vi "Multi RefTriggerScope with digital read.vi"() -> ()   [LabVIEW 2023]
uses:
  RefTriggerApplication/ApplicationCluster.ctl
  <instrlib>/niScope/Controls/niScope trigger source digital.ctl
  <instrlib>/niScope/Controls/niScope trigger slope.ctl
  <instrlib>/niDigital/niDigital.llb/niDigital Export Signal.ctl
  <instrlib>/niDigital/niDigital.llb/niDigital Trigger Digital Edge - Edge.ctl
  <instrlib>/niDigital/niDigital.llb/niDigital Trigger Terminals.ctl
  <instrlib>/niDCPower/nidcpower.llb/niDCPower Export Signal - Signal.ctl
  <instrlib>/niDCPower/nidcpower.llb/niDCPower Wait For Event - Event.ctl
  <instrlib>/niScope/Configure/Trigger/niScope Configure Trigger Digital.vi
  <instrlib>/niDigital/niDigital.llb/niDigital Disable Start Trigger.vi
  <instrlib>/niDigital/niDigital.llb/niDigital Configure Digital Edge Start Trigger.vi
  <instrlib>/niScope/Acquire/Fetch/niScope Fetch.vi
panel:
  out "SMU":dbl[](graph)
  in  "Trigger Through":enum16{"DigitalPattern", "SMU"}(ring)
  in  "Instrument Settings":enum32{"SMU", "Scope", "Digital Pattern"}(tab)
  in  "SMU name":refnum<k15>
  in  "Scope Name 2":refnum<k15>="Scope_5152_C02_S05" caption="Scope  Name(s)"
  in  "Scope Name":refnum<k15>="Scope_5152_C02_S05" caption="Scope  Name(s)"
  in  "Sample Rate":dbl=5000000.0 format="%#.2p"
  in  "Record Length":i32=10000 format="%.0p"
  in  "Reference Position":dbl=50.0 caption="Ref Position" format="%#.1f"
  in  "DigiPat name":refnum<k15>
  in  "pin list":string="SPICLock, SPIData"
  out "Scope":dbl[][](graph)
  out "Digital Data":u32[][](array[numeric])
  out "error out":errorcluster
  in  "error in":errorcluster
  # "SDA"
  # "Other pin"
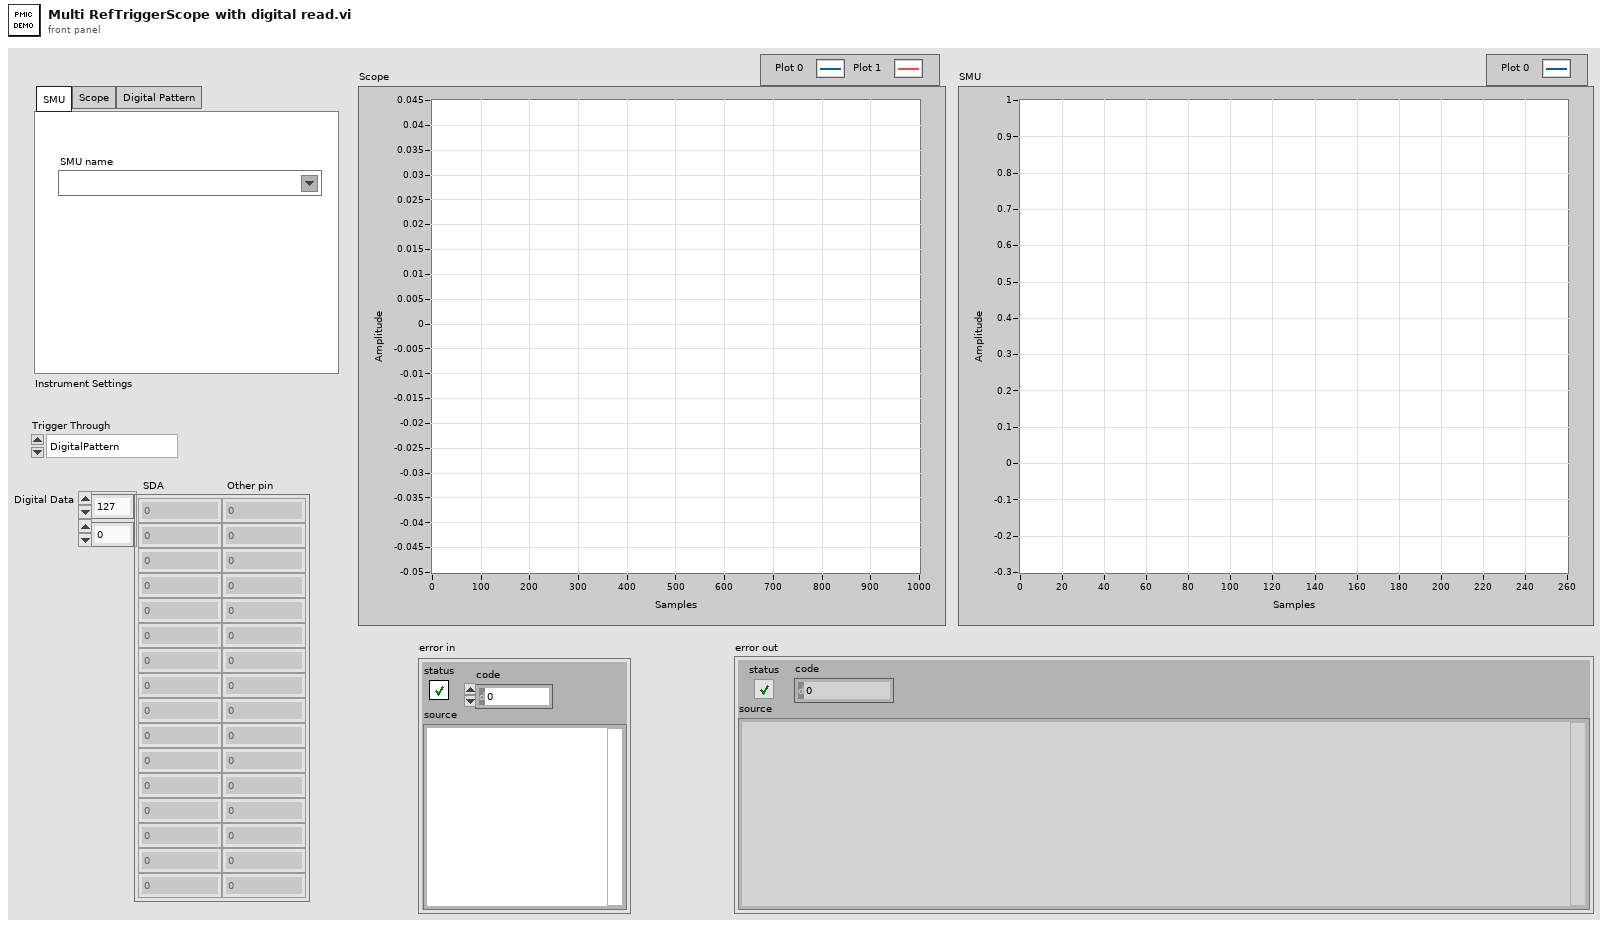
[diagram p1: front panel]
types:
  T1 = typedef "ApplicationCluster.ctl" = cluster{"Scope Name":refnum<k15>, "Scope channel name":string, "DigiPat name":refnum<k15>, "pin list":string, "DigitalWaveformName":string, "DigitalData":u32[][], "SMU name":refnum<k15>, "SMU Channel Name":string, "SMU Sequence Name":string, "Scope wfm":dbl[][], "SMU wfv":dbl[], "Record Length Scope":i32, "Scope Name 2":refnum<k15>, "Scope channel name 2":string}
  T2 = typedef "niScope trigger source digital.ctl" = string
  T3 = typedef "niDigital Trigger Terminals.ctl" = string
  T4 = typedef "niScope trigger slope.ctl" = i32
  T5 = typedef "niDigital Export Signal.ctl" = i32
  T6 = typedef "niDCPower Export Signal - Signal.ctl" = i32
  T7 = typedef "niDigital Trigger Digital Edge - Edge.ctl" = i32
  T8 = typedef "niDCPower Wait For Event - Event.ctl" = i32
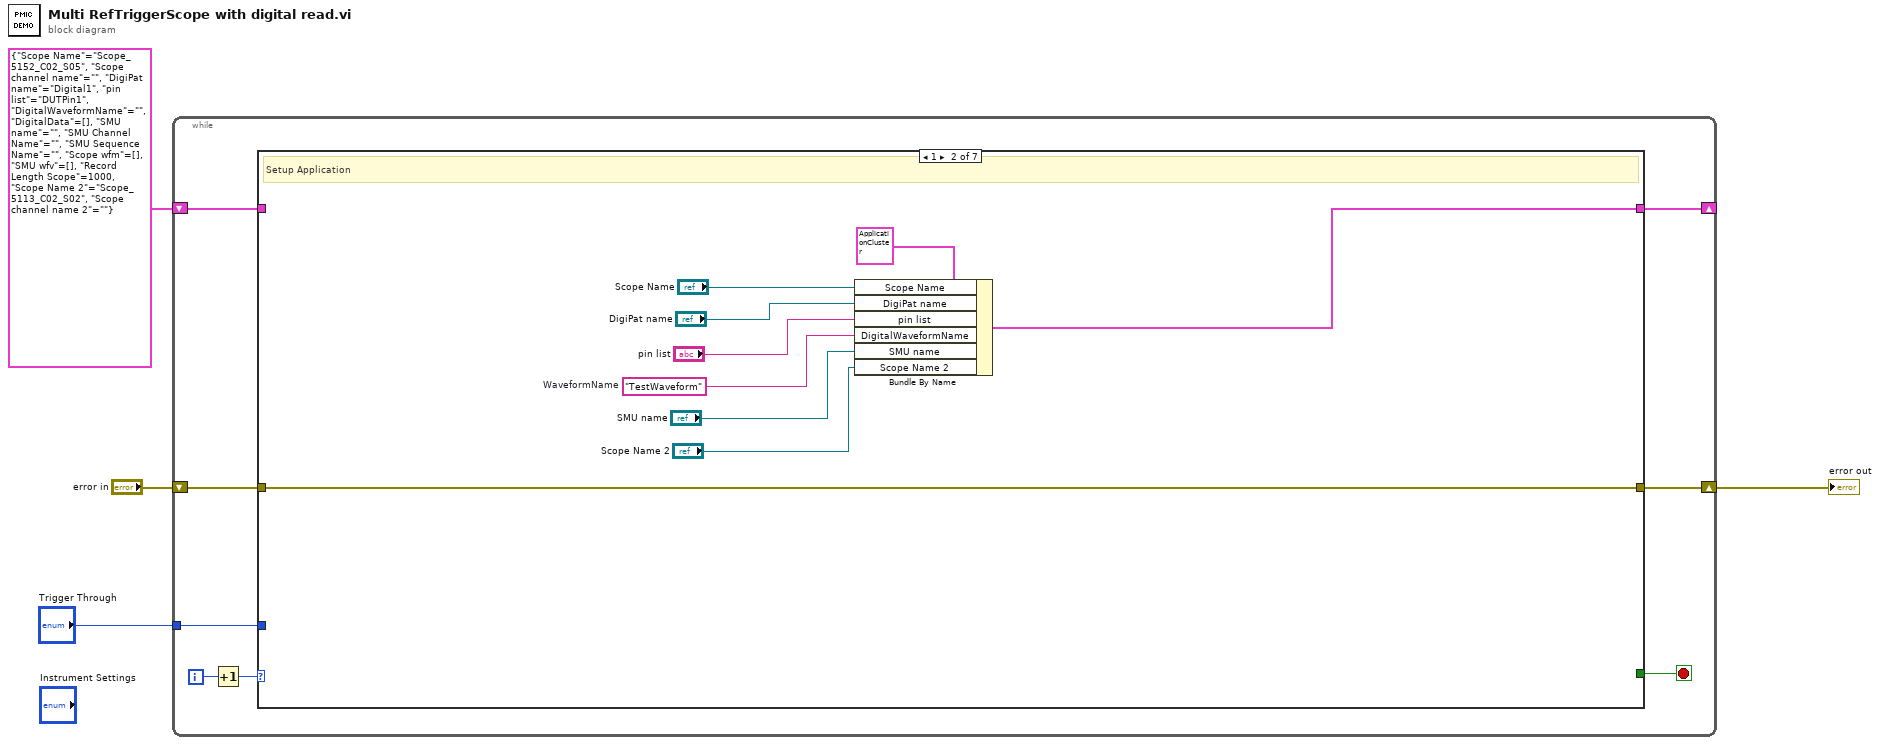
[diagram p0: block diagram]
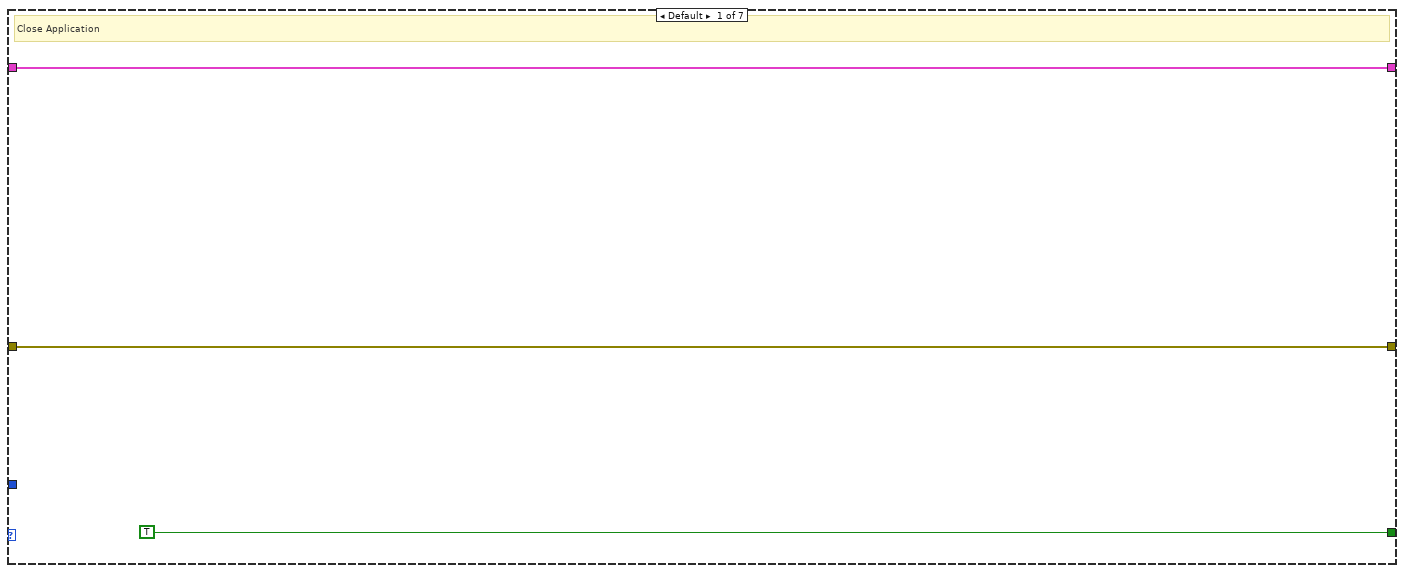
[diagram p2: hidden frame]
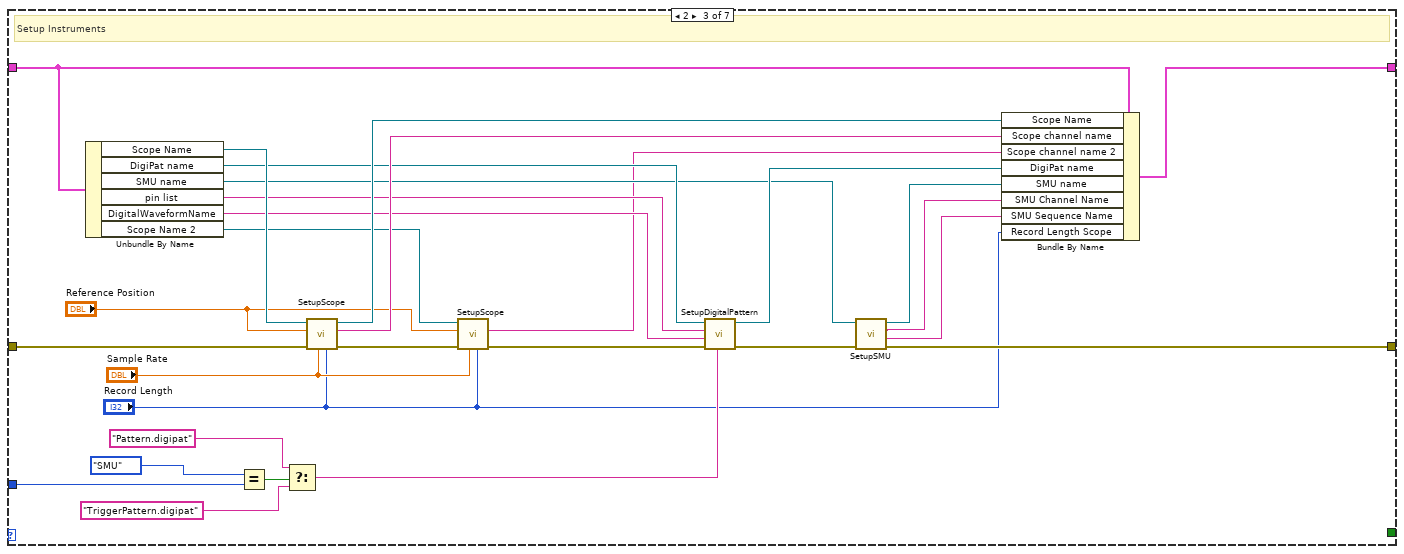
[diagram p3: hidden frame]
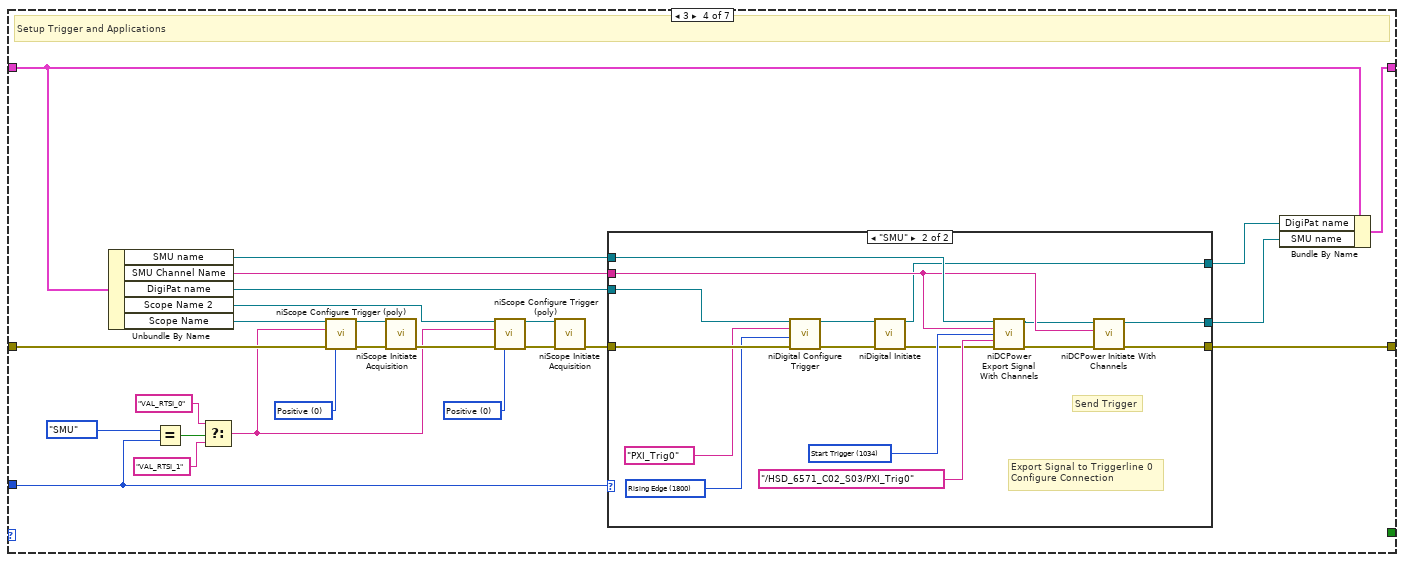
[diagram p4: hidden frame]
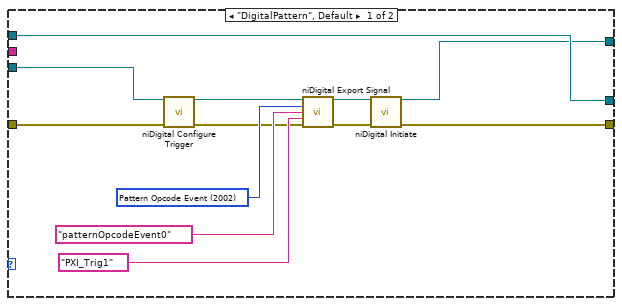
[diagram p5: hidden frame]
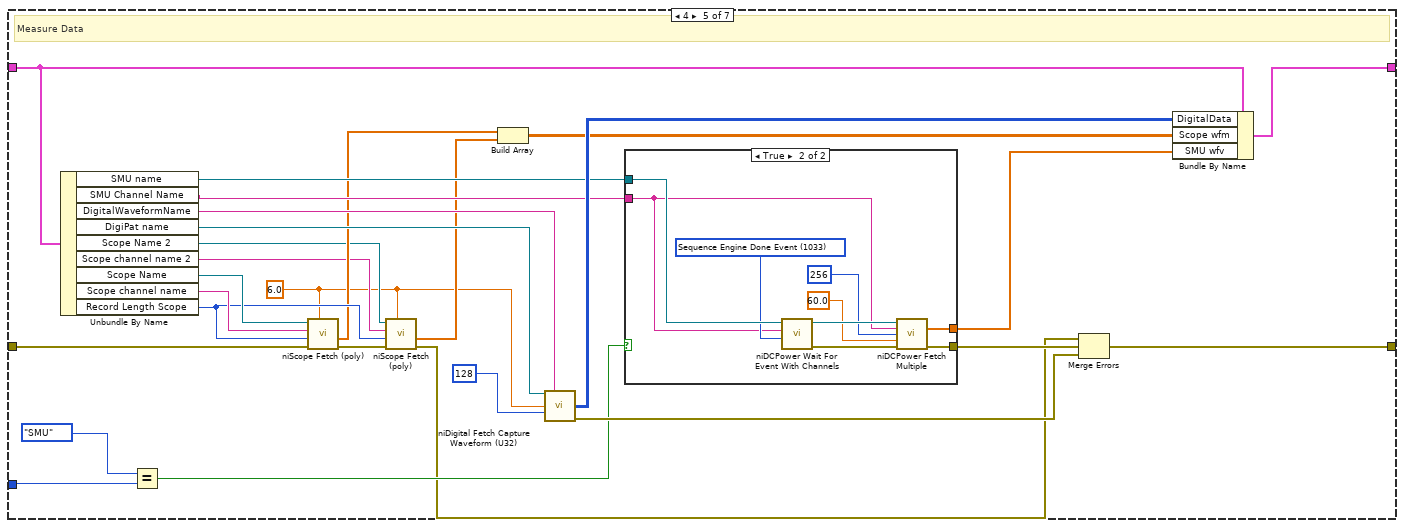
[diagram p6: hidden frame]
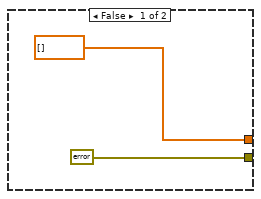
[diagram p7: hidden frame]
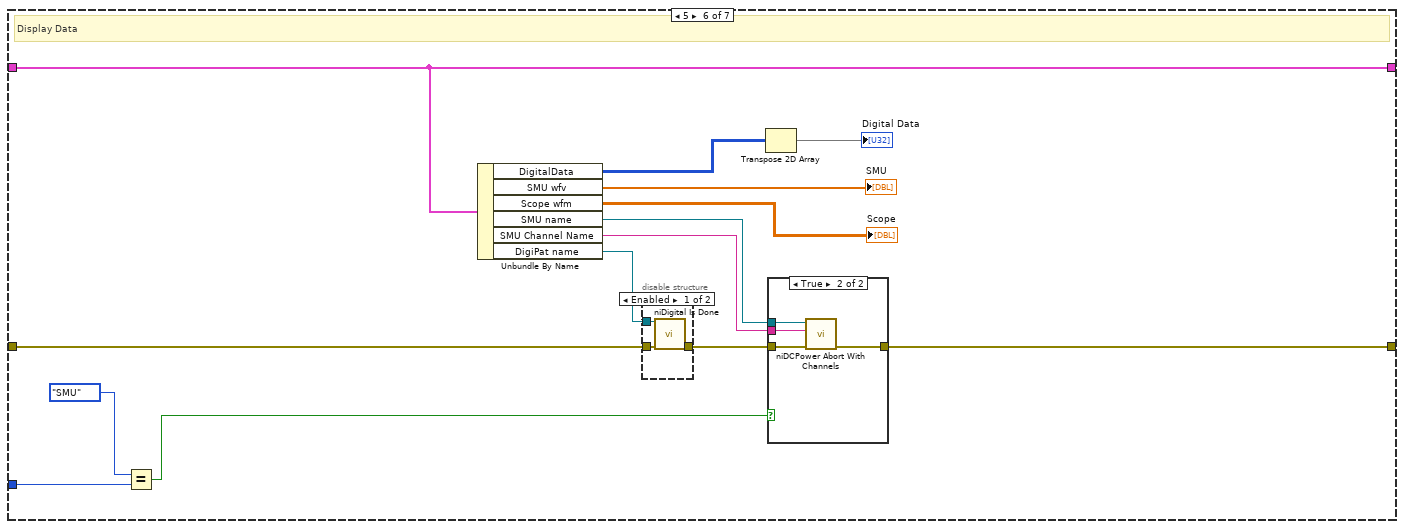
[diagram p8: hidden frame]
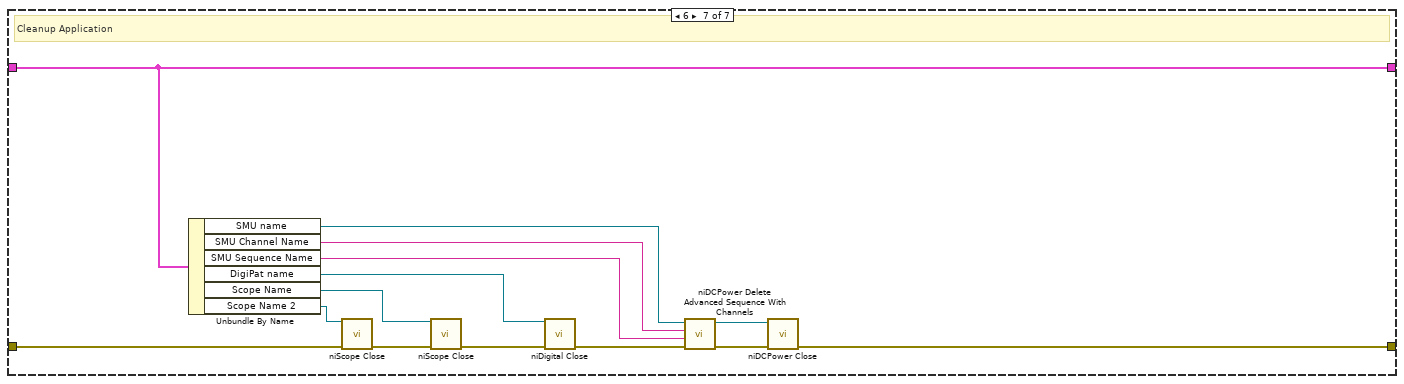
[diagram p11: hidden frame]
diagram:
  n1 = while {
    shift-right: [w12] -> w1
    shift-left: "error in" -> [w11]
    shift-right: [w9] -> _
    shift-left: T1 {"Scope Name"="Scope_5152_C02_S05", "Scope channel name"="", "DigiPat name"="Digital1", "pin list"="DUTPin1", "DigitalWaveformName"="", "DigitalData"=[], "SMU name"="", "SMU Channel Name"="", "SMU Sequence Name"="", "Scope wfm"=[], "SMU wfv"=[], "Record Length Scope"=1000, "Scope Name 2"="Scope_5113_C02_S02", "Scope channel name 2"=""} -> [w8]
    tunnel: "Trigger Through" -> [w5]
    i -> [w6]
    stop <- w10 stop-if-true
    n2 = Increment(x=w6) -> (x+1=w7:i32)
    n3 = case shown="1" w7 {
      tunnel: [w14 w21 w43 w73 w124 w152 w177] -> w12
      tunnel: w11 -> [w14 w21 w53 w66 w133 w156 w169]
      tunnel: [TRUE _ _ _ _ _ _] -> w10
      tunnel: [w13 w22 w49 w77 w129 w158 w180] -> w9
      tunnel: w8 -> [w13 _ w51 w78 w130 w158 w180]
      tunnel: w5 -> [_ _ w37 w63 w119 w151 _]
      frame Default {
        # "Close Application"
      }
      frame 1 {
        w18 = "TestWaveform"  # WaveformName
        # "Setup Application"
        n4 = Bundle By Name(cluster=T1 {"Scope Name"="Scope_5152_C02_S05", "Scope channel name"="", "DigiPat name"="Digital1", "pin list"="DUTPin1", "DigitalWaveformName"="", "DigitalData"=[], "SMU name"="", "SMU Channel Name"="", "SMU Sequence Name"="", "Scope wfm"=[], "SMU wfv"=[], "Record Length Scope"=1000, "Scope Name 2"="Scope_5113_C02_S02", "Scope channel name 2"=""}, "Scope Name"="Scope Name", "DigiPat name"="DigiPat name", "pin list"="pin list", "DigitalWaveformName"=w18, "SMU name"="SMU name", "Scope Name 2"="Scope Name 2") -> (w22:T1)
      }
      frame 2 {
        # "Setup Instruments"
        n5 = Unbundle By Name(w51) -> ("Scope Name"=w52:refnum<k15>, "DigiPat name"=w47:refnum<k15>, "SMU name"=w44:refnum<k15>, "pin list"=w39:string, "DigitalWaveformName"=w38:string, "Scope Name 2"=w27:refnum<k15>)
        n6 = Equal?(x=enum16{"DigitalPattern", "SMU"}."SMU" ("Trigger Through"), y=w37) -> (x = y?=w36:bool)
        n7 = Select(t="Pattern.digipat" ("PatternfileName"), s=w36, f="TriggerPattern.digipat") -> (s? t:f=w33:string)
        n8 = call "SetupScope.vi"("Record Length"="Record Length", "Sample Rate"="Sample Rate", "error in (no error)"=w53, "Reference Position"="Reference Position", "IVI Refnum in"=w52) -> ("error out"=w30:errorcluster, "channel name"=w48:string, "IVI Refnum out"=w50:refnum<k15>)  [unwired: 4 in]
        n9 = call "SetupScope.vi"("Record Length"="Record Length", "Sample Rate"="Sample Rate", "error in (no error)"=w30, "Reference Position"="Reference Position", "IVI Refnum in"=w27) -> ("error out"=w26:errorcluster, "channel name"=w25:string)  [unwired: 4 in, 1 out]
        n10 = call "SetupDigitalPattern.vi"("PatternfileName"=w33, "error in (no error)"=w26, "DigitalWaveformName"=w38, "pin list"=w39, "IVI Refnum in"=w47) -> ("error out"=w45:errorcluster, "IVI Refnum out"=w46:refnum<k15>)  [unwired: 5 in]
        n11 = call "SetupSMU.vi"("error in (no error)"=w45, "IVI Refnum in"=w44) -> ("error out"=w43:errorcluster, "SMU sequence name"=w40:string, "SMU Chanel Name"=w41:string, "instrument handle out"=w42:refnum<k15>)  [unwired: 6 in]
        n12 = Bundle By Name(cluster=w51, "Scope Name"=w50, "Scope channel name"=w48, "Scope channel name 2"=w25, "DigiPat name"=w46, "SMU name"=w42, "SMU Channel Name"=w41, "SMU Sequence Name"=w40, "Record Length Scope"="Record Length") -> (w49:T1)
      }
      frame 3 {
        w59 = T4 0 items=["Positive", "Negative"] ("trigger slope")
        w76 = T4 0 items=["Positive", "Negative"] ("trigger slope")
        # "Setup Trigger and Applications"
        n13 = Unbundle By Name(w78) -> ("SMU name"=w71:refnum<k15>, "SMU Channel Name"=w70:string, "DigiPat name"=w74:refnum<k15>, "Scope Name 2"=w54:refnum<k15>, "Scope Name"=w75:refnum<k15>)
        n14 = Equal?(x=enum16{"DigitalPattern", "SMU"}."SMU" ("Trigger Through"), y=w63) -> (x = y?=w65:bool)
        n15 = Select(t=T2 "VAL_RTSI_0" ("trigger source"), s=w65, f=T2 "VAL_RTSI_1" ("trigger source")) -> (s? t:f=w56:T2)
        n16 = call-poly <instrlib>:"niScope Configure Trigger (poly).vi"("instrument handle"=w75, "trigger slope"=w76, "trigger source"=w56, "error in"=w66) -> ("instrument handle out"=w67:refnum<k15>, "error out"=w68:errorcluster)  [unwired: 10 in]
        n17 = call <instrlib>:"niScope Initiate Acquisition.vi"("instrument handle"=w67, "error in"=w68) -> ("error out"=w58:errorcluster)  [unwired: 12 in, 1 out]
        n18 = call-poly <instrlib>:"niScope Configure Trigger (poly).vi"("instrument handle"=w54, "trigger slope"=w59, "trigger source"=w56, "error in"=w58) -> ("instrument handle out"=w55:refnum<k15>, "error out"=w60:errorcluster)  [unwired: 10 in]
        n19 = call <instrlib>:"niScope Initiate Acquisition.vi"("instrument handle"=w55, "error in"=w60) -> ("error out"=w57:errorcluster)  [unwired: 12 in, 1 out]
        n20 = case shown="\"SMU\"" w63 {
          tunnel: w57 -> [w79 w106]
          tunnel: w74 -> [w82 w105]
          tunnel: [w86 w100] -> w73
          tunnel: [w90 w99] -> w72
          tunnel: w71 -> [w90 w98]
          tunnel: w70 -> [_ w97]
          tunnel: [w83 w92] -> w69
          frame "DigitalPattern", Default {
            w89 = T5 2002 items=["Start Trigger"=2000, "Conditional Jump Trigger"=2001, "Pattern Opcode Event"=2002, "RIO Event"=2004] ("signal")
            n21 = call-poly <instrlib>:"niDigital Configure Trigger.vi"("instrument handle"=w82, "error in"=w79) -> ("instrument handle out"=w81:refnum<k15>, "error out"=w80:errorcluster)  [unwired: 12 in]
            n22 = call <instrlib>:"niDigital Export Signal.vi"("instrument handle"=w81, "signal"=w89, "signal ID"="patternOpcodeEvent0", "output terminal"="PXI_Trig1", "error in"=w80) -> ("instrument handle out"=w84:refnum<k15>, "error out"=w85:errorcluster)  [unwired: 9 in]
            n23 = call <instrlib>:"niDigital Initiate.vi"("instrument handle"=w84, "error in"=w85) -> ("instrument handle out"=w83:refnum<k15>, "error out"=w86:errorcluster)  [unwired: 12 in]
          }
          frame "SMU" {
            w102 = T6 1034 items=["Source Complete Event"=1030, "Measure Complete Event"=1031, "Sequence Iteration Complete Event"=1032, "Sequence Engine Done Event"=1033, "Pulse Complete Event"=1051, "Ready For Pulse Trigger Event"=1052, "Start Trigger"=1034, "Source Trigger"=1035, "Measure Trigger"=1036, "Sequence Advance Trigger"=1037, "Pulse Trigger"=1053] ("signal")
            w104 = T7 1800 items=["Rising Edge"=1800, "Falling Edge"=1801] ("edge")
            # "Send Trigger"
            # "Export Signal to Triggerline 0\nConfigure Connection"
            n24 = call-poly <instrlib>:"niDigital Configure Trigger.vi"("instrument handle"=w105, "source"=T3 "PXI_Trig0", "edge"=w104, "error in"=w106) -> ("instrument handle out"=w95:refnum<k15>, "error out"=w96:errorcluster)  [unwired: 10 in]
            n25 = call <instrlib>:"niDigital Initiate.vi"("instrument handle"=w95, "error in"=w96) -> ("instrument handle out"=w92:refnum<k15>, "error out"=w94:errorcluster)  [unwired: 12 in]
            n26 = call <instrlib>:"niDCPower Export Signal With Channels.vi"("instrument handle"=w98, "channel name"=w97, "signal"=w102, "output terminal"=tag "/HSD_6571_C02_S03/PXI_Trig0", "error in (no error)"=w94) -> ("instrument handle out"=w91:refnum<k15>, "error out"=w93:errorcluster)  [unwired: 9 in]
            n27 = call <instrlib>:"niDCPower Initiate With Channels.vi"("error in (no error)"=w93, "channel name"=w97, "instrument handle"=w91) -> ("error out"=w100:errorcluster, "instrument handle out"=w99:refnum<k15>)  [unwired: 7 in]
          }
        }
        n28 = Bundle By Name(cluster=w78, "DigiPat name"=w69, "SMU name"=w72) -> (w77:T1)
      }
      frame 4 {
        w107 = 6.0 ("timeout")
        # "Measure Data"
        n29 = Unbundle By Name(w130) -> ("SMU name"=w127:refnum<k15>, "SMU Channel Name"=w126:string, "DigitalWaveformName"=w125:string, "DigiPat name"=w121:refnum<k15>, "Scope Name 2"=w109:refnum<k15>, "Scope channel name 2"=w108:string, "Scope Name"=w132:refnum<k15>, "Scope channel name"=w131:string, "Record Length Scope"=w113:i32)
        n30 = Equal?(x=enum16{"DigitalPattern", "SMU"}."SMU" ("Trigger Through"), y=w119) -> (x = y?=w118:bool)
        n31 = call-poly <instrlib>:"niScope Fetch (poly).vi"("timeout"=w107, "error in"=w133, "numSamples"=w113, "channels"=w131, "instrument handle"=w132) -> ("error out"=w114:errorcluster, "wfm"=w112:dbl[])  [unwired: 3 in, 2 out]
        n32 = call-poly <instrlib>:"niScope Fetch (poly).vi"("timeout"=w107, "error in"=w114, "numSamples"=w113, "channels"=w108, "instrument handle"=w109) -> ("error out"=w115:errorcluster, "wfm"=w111:dbl[])  [unwired: 3 in, 2 out]
        n33 = Build Array(w112, w111) -> (w110:dbl[][])
        n34 = call <instrlib>:"niDigital Fetch Capture Waveform (U32).vi"("instrument handle"=w121, "waveform name"=w125, "timeout (s)"=w107, "samples to read"=128) -> ("data"=w128:u32[][], "error out"=w122:errorcluster)  [unwired: 9 in, 1 out]
        n35 = case shown="True" w118 {
          tunnel: w127 -> [_ w142]
          tunnel: w126 -> [_ w140]
          tunnel: [errorcluster {"status"=FALSE, "code"=0, "source"=""} ("error out") w139] -> w123
          tunnel: [dbl[] [] ("voltage measurements") w138] -> w116
          frame False {
          }
          frame True {
            w141 = T8 1033 items=["Source Complete Event"=1030, "Measure Complete Event"=1031, "Sequence Iteration Complete Event"=1032, "Sequence Engine Done Event"=1033, "Pulse Complete Event"=1051, "Ready For Pulse Trigger Event"=1052] ("event")
            n36 = call <instrlib>:"niDCPower Wait For Event With Channels.vi"("event"=w141, "channel name"=w140, "instrument handle"=w142) -> ("error out"=w143:errorcluster, "instrument handle out"=w144:refnum<k15>)  [unwired: 7 in]
            n37 = call <instrlib>:"niDCPower Fetch Multiple.vi"("instrument handle"=w144, "channel name"=w140, "count (1)"=256 ("numSamples"), "timeout (1.0)"=60.0, "error in (no error)"=w143) -> ("voltage measurements"=w138:dbl[], "error out"=w139:errorcluster)  [unwired: 5 in, 4 out]
          }
        }
        n38 = Merge Errors(w115, w123, w122) -> (w124:errorcluster)
        n39 = Bundle By Name(cluster=w130, "DigitalData"=w128, "Scope wfm"=w110, "SMU wfv"=w116) -> (w129:T1)
      }
      frame 5 {
        # "Display Data"
        n40 = Equal?(x=enum16{"DigitalPattern", "SMU"}."SMU" ("Trigger Through"), y=w151) -> (x = y?=w150:bool)
        n41 = Unbundle By Name(w158) -> ("DigitalData"=w146:u32[][], "SMU wfv"=→"SMU":dbl[], "Scope wfm"=→"Scope":dbl[][], "SMU name"=w153:refnum<k15>, "SMU Channel Name"=w154:string, "DigiPat name"=w157:refnum<k15>)
        n42 = disable-structure shown="Enabled" {
          disable-tunnel: w157 -> [w166 _]
          disable-tunnel: w156 -> [w165 w167]
          disable-tunnel: [w164 w167] -> w155
          frame Enabled {
            n43 = call <instrlib>:"niDigital Is Done.vi"("instrument handle"=w166, "error in"=w165) -> ("error out"=w164:errorcluster)  [unwired: 11 in, 2 out]
          }
          frame Disabled {
          }
        }
        n44 = Transpose 2D Array(2D array=w146) -> (transposed array=→"Digital Data":u32[][])
        n45 = case shown="True" w150 {
          tunnel: w155 -> [w159 w163]
          tunnel: w154 -> [_ w162]
          tunnel: w153 -> [_ w161]
          tunnel: [w159 w160] -> w152
          frame False {
          }
          frame True {
            n46 = call <instrlib>:"niDCPower Abort With Channels.vi"("error in (no error)"=w163, "channel name"=w162, "instrument handle"=w161) -> ("error out"=w160:errorcluster)  [unwired: 7 in, 1 out]
          }
        }
      }
      frame 6 {
        # "Cleanup Application"
        n47 = Unbundle By Name(w180) -> ("SMU name"=w173:refnum<k15>, "SMU Channel Name"=w172:string, "SMU Sequence Name"=w171:string, "DigiPat name"=w178:refnum<k15>, "Scope Name"=w181:refnum<k15>, "Scope Name 2"=w170:refnum<k15>)
        n48 = call <instrlib>:"niScope Close.vi"("instrument handle"=w170, "error in"=w169) -> ("error out"=w168:errorcluster)  [unwired: 13 in]
        n49 = call <instrlib>:"niScope Close.vi"("instrument handle"=w181, "error in"=w168) -> ("error out"=w179:errorcluster)  [unwired: 13 in]
        n50 = call <instrlib>:"niDigital Close.vi"("instrument handle"=w178, "error in"=w179) -> ("error out"=w176:errorcluster)  [unwired: 13 in]
        n51 = call <instrlib>:"niDCPower Delete Advanced Sequence With Channels.vi"("error in (no error)"=w176, "sequence name"=w171, "channel name"=w172, "instrument handle"=w173) -> ("error out"=w175:errorcluster, "instrument handle out"=w174:refnum<k15>)  [unwired: 6 in]
        n52 = call <instrlib>:"niDCPower Close.vi"("error in (no error)"=w175, "instrument handle"=w174) -> ("error out"=w177:errorcluster)  [unwired: 9 in]
      }
    }
  }
  "error out" <- w1
